vi "POT.vi"() -> ()   [LabVIEW 2013]
panel:
  out "POT":dbl
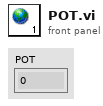
[diagram p1: front panel]
diagram:
